vi "GetServerDetPars.vi"   [LabVIEW 2014]
uses:
  globals/DetectorGlobals.vi
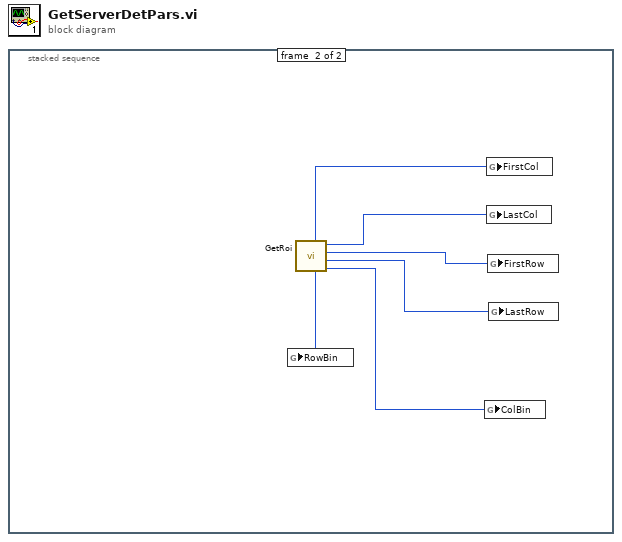
[diagram p0: block diagram]
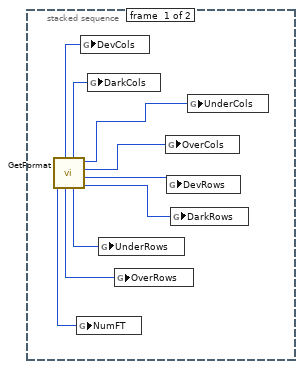
[diagram p2: hidden frame]
diagram:
  n1 = stacked-sequence {
    frame #0 {
      n2 = call "GetFormat.vi"() -> ("NPdark"=w4:i32, "NPtotal"=w7:i32, "NSoverscan"=w6:i32, "NSunderscan"=w5:i32, "NPunderscan"=w3:i32, "NSdark"=w8:i32, "NPoverscan"=w2:i32, "NStotal"=w9:i32, "NPframetransfer"=w1:i32)  [unwired: 3 in]
      n3 = global write "DetectorGlobals.vi" "NumFT"(w1) -> ()
      n4 = global write "DetectorGlobals.vi" "DevCols"(w9) -> ()
      n5 = global write "DetectorGlobals.vi" "DarkCols"(w8) -> ()
      n6 = global write "DetectorGlobals.vi" "UnderRows"(w3) -> ()
      n7 = global write "DetectorGlobals.vi" "OverRows"(w2) -> ()
      n8 = global write "DetectorGlobals.vi" "OverCols"(w6) -> ()
      n9 = global write "DetectorGlobals.vi" "DevRows"(w7) -> ()
      n10 = global write "DetectorGlobals.vi" "DarkRows"(w4) -> ()
      n11 = global write "DetectorGlobals.vi" "UnderCols"(w5) -> ()
    }
    frame #1 {
      n12 = call "GetRoi.vi"() -> ("FirstCol"=w15:i32, "RowBin"=w10:i32, "LastCol"=w14:i32, "FirstRow"=w13:i32, "LastRow"=w12:i32, "ColBin"=w11:i32)  [unwired: 1 in]
      n13 = global write "DetectorGlobals.vi" "RowBin"(w10) -> ()
      n14 = global write "DetectorGlobals.vi" "ColBin"(w11) -> ()
      n15 = global write "DetectorGlobals.vi" "FirstCol"(w15) -> ()
      n16 = global write "DetectorGlobals.vi" "LastCol"(w14) -> ()
      n17 = global write "DetectorGlobals.vi" "FirstRow"(w13) -> ()
      n18 = global write "DetectorGlobals.vi" "LastRow"(w12) -> ()
    }
  }
